vi "String.Replace Subset with Variant Attribute.vi"(7 "Vars":variant, 11 "Data In":string) -> (2 "error out":errorcluster, 3 "Data Out":string)   [LabVIEW 2024]
uses:
  Errors/Error.Error Code List.ctl
  Errors.lvlib
panel:
  in  "Test":bool
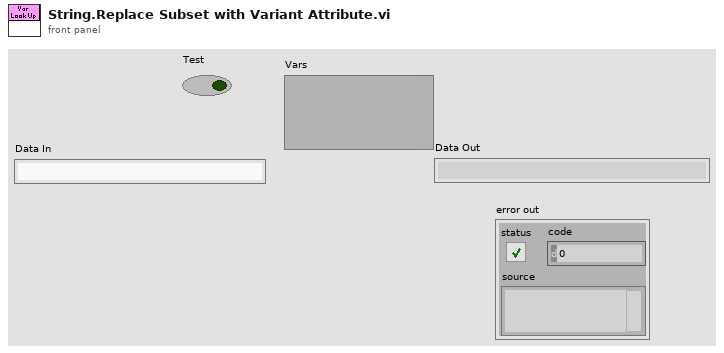
[diagram p1: front panel]
types:
  T1 = typedef "EQMF.lvlib/Errors.lvlib/Error.Error Code List.ctl" = i32
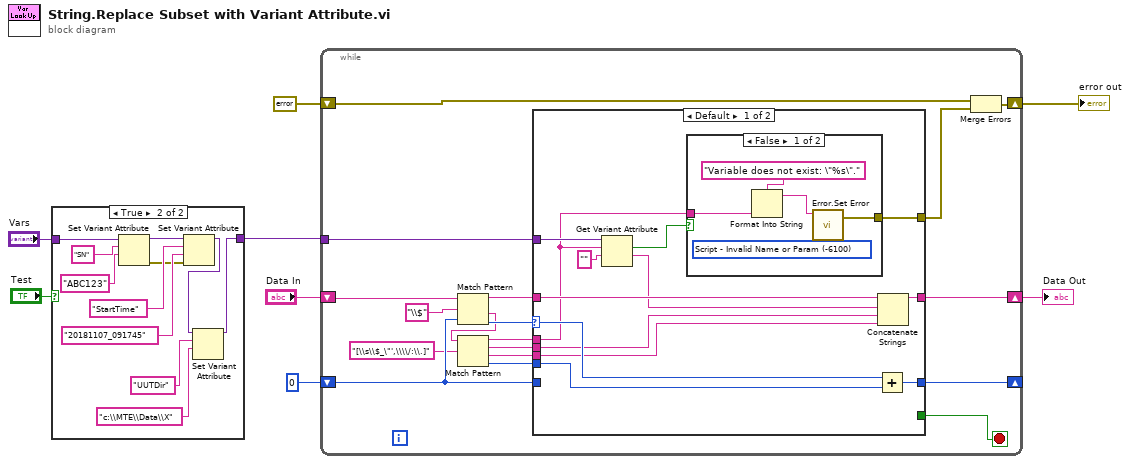
[diagram p0: block diagram]
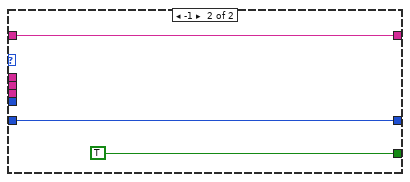
[diagram p4: hidden frame]
diagram:
  n1 = case shown="True" "Test" {
    tunnel: "Vars" -> [w9 w20]
    tunnel: [w9 w15] -> w4
    frame False {
    }
    frame True {
      n2 = Set Variant Attribute(Variant=w20, name="SN", value="ABC123" ("name")) -> (Variant out=w11:variant, error out=w12:errorcluster)  [unwired: 1 in, 1 out]
      n3 = Set Variant Attribute(Variant=w11, name="StartTime", value="20181107_091745" ("name"), error in=w12) -> (Variant out=w10:variant)  [unwired: 2 out]
      n4 = Set Variant Attribute(Variant=w10, name="UUTDir", value="c:\\MTE\\Data\\X" ("name")) -> (Variant out=w15:variant)  [unwired: 1 in, 2 out]
    }
  }
  n5 = while {
    tunnel: w4 -> [w26]
    shift-right: [w31] -> w6
    shift-left: "Data In" -> [w38]
    shift-right: [w28] -> _
    shift-left: 0 -> [w29]
    shift-right: [w23] -> w2
    shift-left: errorcluster {"status"=FALSE, "code"=0, "source"=""} ("error out") -> [w22]
    stop <- w30 stop-if-true
    n6 = Match Pattern(string=w38, regular expression="\\$", offset (0)=w29) -> (before substring=w32:string, after substring=w34:string, offset past match=w36:i32)  [unwired: 1 out]
    n7 = Match Pattern(string=w34, regular expression="[\\s\\$_\"',\\\\/:\\.]") -> (before substring=w35:string, match substring=w25:string, after substring=w33:string, offset past match=w27:i32)  [unwired: 1 in]
    n8 = case shown="Default" w36 {
      selector: w36 -> [w50 _]
      tunnel: w35 -> [w40 _]
      tunnel: w33 -> [w42 _]
      tunnel: w32 -> [w45 w59]
      tunnel: [w46 w59] -> w31
      tunnel: [_ TRUE] -> w30
      tunnel: w29 -> [_ w57]
      tunnel: [w51 w57] -> w28
      tunnel: w27 -> [w49 _]
      tunnel: w26 -> [w48 _]
      tunnel: w25 -> [w43 _]
      tunnel: [w39 _] -> w21
      frame Default {
        n9 = Get Variant Attribute(Variant=w48, name=w40, default value (empty Variant)="") -> (found=w41:bool, value=w44:string)  [unwired: 1 in, 2 out]
        n10 = case shown="False" w41 {
          tunnel: w40 -> [w55 _]
          tunnel: [w52 _] -> w39
          frame False {
            w53 = T1 -6100 items=["No Error"=0, "Abort"=-2, "Misc"=-5000, "Fixture Error"=-5100, "File IO - General"=-5200, "FIle IO - Config Error"=-5201, "Instrument - General"=-5300, "Instrument - Serial Com"=-5301, "Instrument - Camera"=-5302, "Instrument - PS"=-5303, "Instrument - Oscilloscope"=-5304, "Instrument - Function Gen"=-5305, "Instrument - Load"=-5306, "Instrument - Meter"=-5307, "Instrument - Power Control"=-5308, "Instrument - Motion"=-5309, "Instrument - RF"=-5310, "System Exe"=-5400, "Image Processing"=-5500, "Communication"=-5600, "Script - Syntax Error"=-6000, "Script - Invalid Name or Param"=-6100, "Script - Timeout"=-6200, "Invalid Data"=-6300, "FW Update Error"=-6500] ("Std Code")
            n11 = Format Into String(format string="Variable does not exist: \"%s\".", w55) -> (resulting string=w54:string)  [unwired: 2 in, 1 out]
            n12 = call "Error.Set Error.vi"("Std Code"=w53, "Desc"=w54) -> ("error out"=w52:errorcluster)  [unwired: 5 in]
          }
          frame True {
          }
        }
        n13 = Add(x=w50, y=w49) -> (x+y=w51:i32)
        n14 = Concatenate Strings(w45, w44, w43, w42) -> (w46:string)
      }
      frame -1 {
      }
    }
    n15 = Merge Errors(w22, w21) -> (w23:errorcluster)
  }
  "Data Out" <- w6
  "error out" <- w2
